vi "PH_GUI.Manager Open.vi"(0 "i ref in":refnum<vi>, 5 "error in":errorcluster) -> (14 "i ref out":refnum<vi>, 19 "error out":errorcluster)   [LabVIEW 2014, in "PH_Common.lvlib"]
doc: "This VI has typically to be set in the constructor of a class. In case of \"Manager File Path\" is not empty or \"N/A\", it tries to read the the last current position of the GUI from a xml-file at the place and file name wired."
uses:
  PH_Common.lvlib
  <vilib>/Utility/xml.llb/Read From XML File(array).vi
  CS_Core/CSObj/CSObj.lvlib
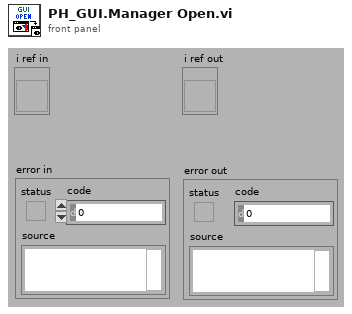
[diagram p1: front panel]
types:
  T1 = typedef "LVRectTypeDef.ctl" = cluster{"Left":i16, "Top":i16, "Right":i16, "Bottom":i16}
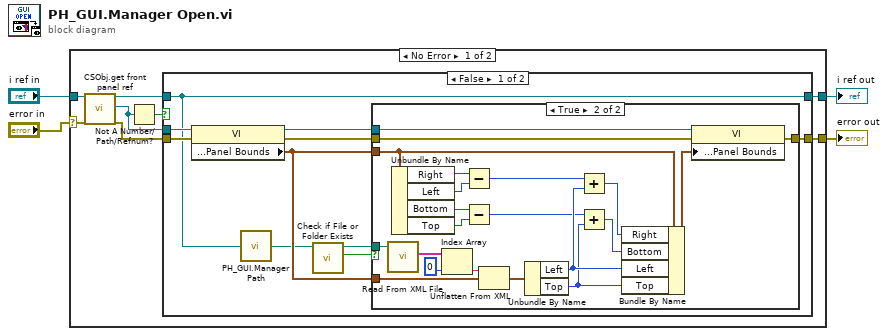
[diagram p0: block diagram]
diagram:
  n1 = case shown="No Error" "error in" {
    selector: "error in" -> [w12 w47]
    tunnel: [w10 w47] -> w4
    tunnel: [w5 w46] -> w3
    tunnel: "i ref in" -> [w11 w46]
    frame No Error {
      n2 = call "CSObj.get front panel ref.vi"("i ref in"=w11, "error in (no error)"=w12) -> ("i ref out"=w6:refnum<vi>, "frontPanelRef"=w8:refnum<vi>, "error out"=w9:errorcluster)  [unwired: 15 in]
      n3 = Not A Number/Path/Refnum?(number/path/refnum=w8) -> (NaN/Path/Refnum?=w7:bool)
      n4 = case shown="False" w7 {
        tunnel: [w21 w45] -> w10
        tunnel: w9 -> [w20 w45]
        tunnel: w8 -> [w18 _]
        tunnel: w6 -> [w15 w44]
        tunnel: [w15 w44] -> w5
        frame False {
          n5 = property class="VI"(reference=w18, error in=w20) -> (error out=w19:errorcluster, "Front Panel Window:Panel Bounds"=w16:T1)  [unwired: 1 out]
          n6 = call "PH_GUI.Manager Path.vi"("i ref in"=w15) -> ("GUI Manager Path"=w14:path)
          n7 = call <vilib>:"Check if File or Folder Exists.vi"("path"=w14) -> ("file or folder exists?"=w13:bool, "dup path"=w17:path)  [unwired: 8 in, 1 out]
          n8 = case shown="True" w13 {
            tunnel: [w22 w43] -> w21
            tunnel: w19 -> [w22 w41]
            tunnel: w16 -> [_ w38]
            tunnel: w18 -> [_ w37]
            tunnel: w17 -> [_ w36]
            tunnel: w16 -> [_ w33]
            frame False {
            }
            frame True {
              n9 = call-poly <vilib>:"Read From XML File.vi"("XML File Path"=w36) -> ("XML Elements"=w42:string[])  [unwired: 8 in, 2 out]
              n10 = Unbundle By Name(w33) -> ("Right"=w32:i16, "Left"=w31:i16, "Bottom"=w30:i16, "Top"=w29:i16)
              n11 = Index Array(array=w42, index=0) -> (element=w39:string)
              n12 = Subtract(x=w32, y=w31) -> (x-y=w28:i16)
              n13 = Subtract(x=w30, y=w29) -> (x-y=w23:i16)
              n14 = Unflatten From XML(xml string=w39, type=w38) -> (value=w35:T1)  [unwired: 1 in, 1 out]
              n15 = Unbundle By Name(w35) -> ("Left"=w27:i16, "Top"=w24:i16)
              n16 = Add(x=w28, y=w27) -> (x+y=w26:i16)
              n17 = Add(x=w23, y=w24) -> (x+y=w25:i16)
              n18 = Bundle By Name(cluster=w33, "Right"=w26, "Bottom"=w25, "Left"=w27, "Top"=w24) -> (w34:T1)
              n19 = property class="VI"(reference=w37, error in=w41, "Front Panel Window:Panel Bounds"=w34) -> (error out=w43:errorcluster)  [unwired: 1 out]
            }
          }
        }
        frame True {
        }
      }
    }
    frame Error {
    }
  }
  "error out" <- w4
  "i ref out" <- w3
